vi "Cluster to Variant Attributes.vi"(8 "error in (no error)":errorcluster, 11 "Cluster in":refnum<vi>) -> (0 "error out":errorcluster, 3 "Variant out":variant)   [LabVIEW 2020, in "SQSnobFit Control Panel.lvlib"]
doc: "Converts a cluster with named elements to a variant with attributes named after the named elements, containing the same values as the named elements. Unnamed cluster elements are ignored."
uses:
  SQSnobFit Control Panel.lvlib
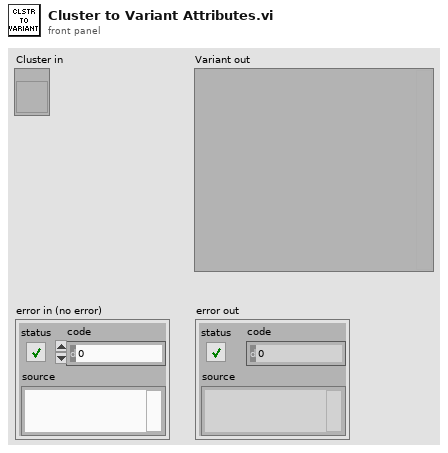
[diagram p1: front panel]
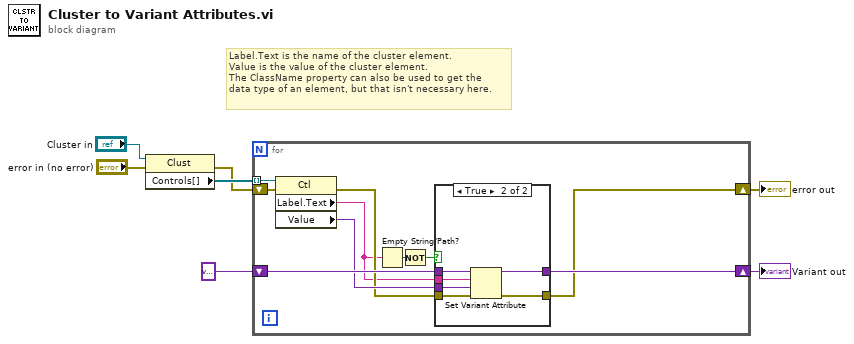
[diagram p0: block diagram]
diagram:
  # "Label.Text is the name of the cluster element.\nValue is the value of the cluster element.\nThe ClassName property can also be used to get the\ndata type of an element, but that isn't necessary here."
  n1 = property on="Property Node" class="Clust"(reference="Cluster in", error in="error in (no error)") -> (error out=w4:errorcluster, "Controls[]"=w7:refnum<vi>[])  [unwired: 1 out]
  n2 = for {
    tunnel: w7 -> [w17] mode=indexing
    shift-right: [w14] -> w5
    shift-left: variant -> [w16]
    shift-right: [w11] -> w3
    shift-left: w4 -> [w13]
    n3 = property class="Ctl"(reference=w17, error in=w13) -> (error out=w12:errorcluster, "Label.Text"=w9:string, "Value"=w15:variant)  [unwired: 1 out]
    n4 = Empty String/Path?(string/path=w9) -> (empty?=w10:bool)
    n5 = Not(x=w10) -> (.not. x?=w8:bool)
    n6 = case shown="True" w8 {
      tunnel: w16 -> [w19 w25]
      tunnel: w15 -> [_ w24]
      tunnel: [w19 w23] -> w14
      tunnel: w12 -> [w18 w22]
      tunnel: [w18 w21] -> w11
      tunnel: w9 -> [_ w20]
      frame False {
        # "Ignore unnamed\nelements"
      }
      frame True {
        n7 = Set Variant Attribute(Variant=w25, name=w20, value=w24, error in=w22) -> (Variant out=w23:variant, error out=w21:errorcluster)  [unwired: 1 out]
      }
    }
  }
  "Variant out" <- w5
  "error out" <- w3
